vi "XY Graph Get Head & Tail Fraction from Cursors.vi"(5 "Active Plot Index":i32, 6 "Use Cursors":bool, 7 "XYGraph in":T1, 8 "error in (no error)":errorcluster, 9 "Tail Fraction":dbl, 10 "Head Fraction":dbl, 11 "Plot in (Default: Use XY Graph refnum & Plot Id)":cluster{"X Array":dbl[], "Y Array":dbl[]}) -> (0 "error out":errorcluster, 1 "Tail Fraction":dbl, 2 "Head Fraction":dbl, 3 "Plot out":cluster{"X Array":dbl[], "Y Array":dbl[]}, 4 "Plot Name":string)   [LabVIEW 2021, in "XY Graph Add-Ons.lvlib"]
doc: "Computes the fractional location of the head and tail fraction from the <B>HE</B> and <B>TS</B> cursors locations.\n\nIf one (or both) of the cursors is missing, keep the existing values."
uses:
  XY Graph Add-Ons.lvlib
  XY Graph Refnum.ctl
  Strings/Strings.lvlib
  Sound/Sound.lvlib
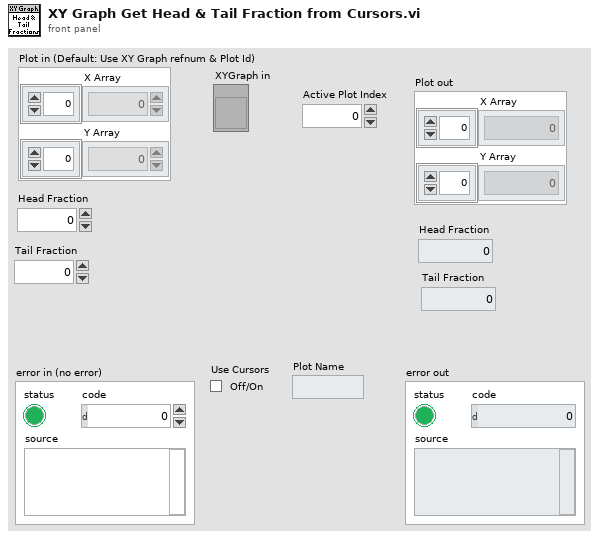
[diagram p1: front panel]
types:
  T1 = typedef "XY Graph Add-Ons.lvlib/XY Graph Refnum.ctl" = refnum<vi>
  T2 = typedef "LVCursorListTypeDef.ctl" = cluster{"Name":string, "Color":u32, "Style":u8, "Point Style":u8, "Name Visible":bool, "Allow Drag":bool, "Cursor Mode":u32, "Plot":i32, "Index":i32, "Position":cluster{"X":dbl, "Y":dbl}, "X Scale":u32, "Y Scale":u32, "Watch Plots":i32[], "Watch All Plots":bool, "Plot Area":i32, "Label Offset":cluster{"X":dbl, "Y":dbl}}[]
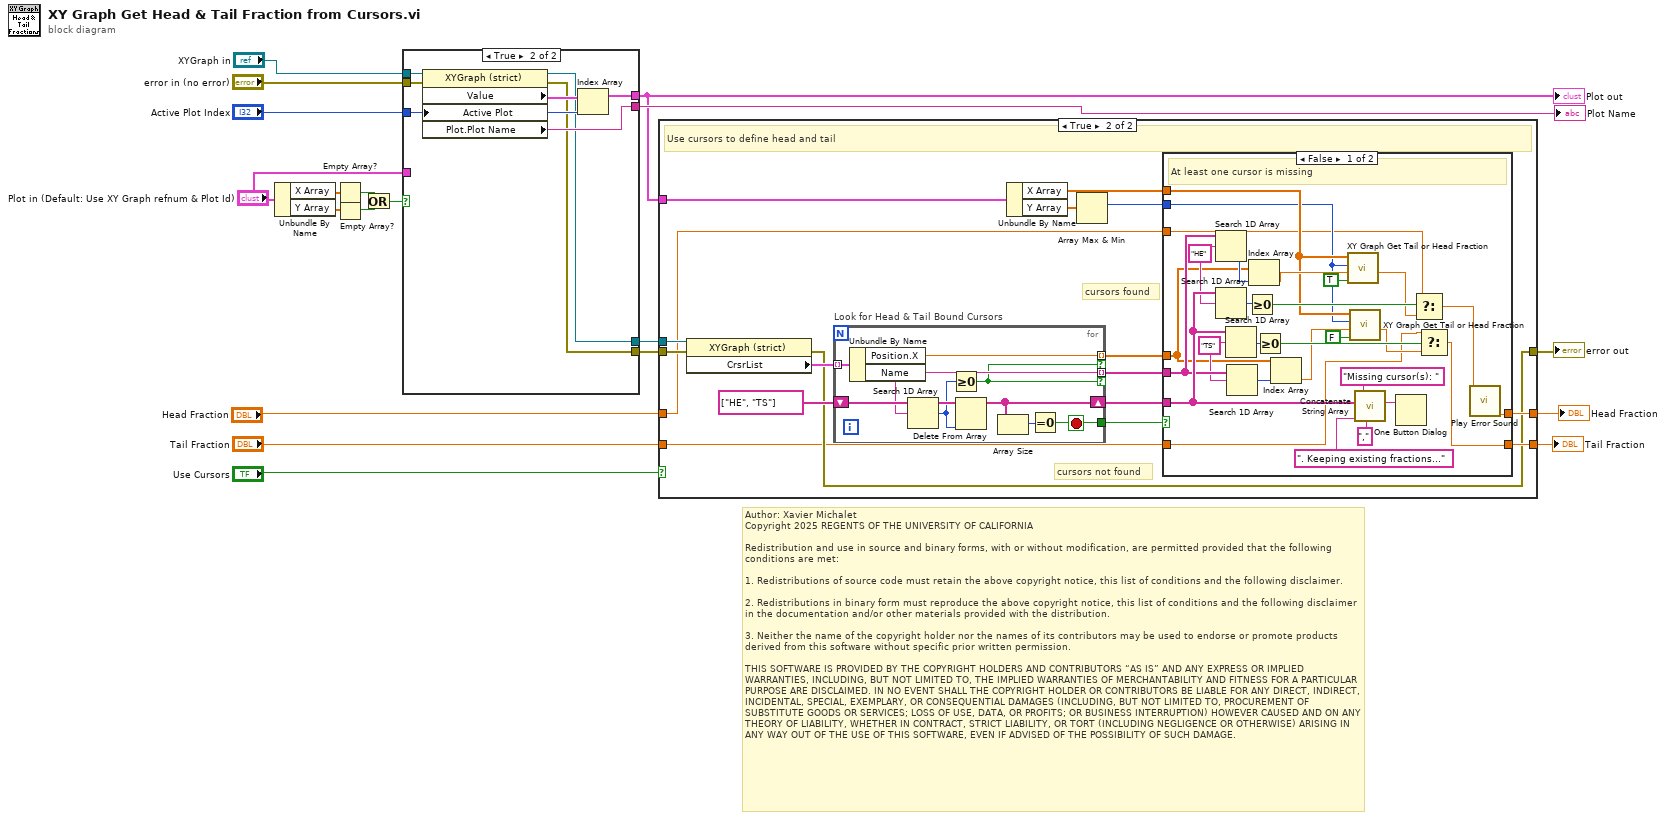
[diagram p0: block diagram]
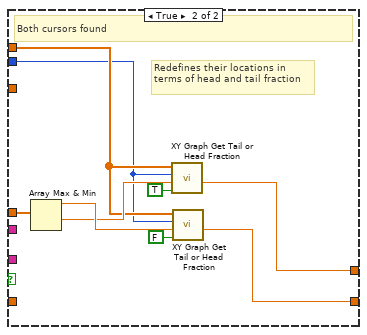
[diagram p4: hidden frame]
diagram:
  # "Author: Xavier Michalet\nCopyright 2025 REGENTS OF THE UNIVERSITY OF CALIFORNIA\n\nRedistribution and use in source and binary forms, with or without modification, are permitted provided that the following conditions are met:\n\n1. Redistributions of source code must retain the above copyright notice, this list of conditions and the following disclaimer.\n\n2. Redistributions in binary form must reproduce the above copyright notice, this list of conditions and the following disclaimer in the documentation and/or other materials provided with the distribution.\n\n3. Neither the name of the copyright holder nor the names of its contributors may be used to endorse or promote products derived from this software without specific prior written permission.\n\nTHIS SOFTWARE IS PROVIDED BY THE COPYRIGHT HOLDERS AND CONTRIBUTORS “AS IS” AND ANY EXPRESS OR IMPLIED WARRANTIES, INCLUDING, BUT NOT LIMITED TO, THE IMPLIED WARRANTIES OF MERCHANTABILITY AND FITNESS FOR A PARTICULAR PURPOSE ARE DISCLAIMED. IN NO EVENT SHALL THE COPYRIGHT HOLDER OR CONTRIBUTORS BE LIABLE FOR ANY DIRECT, INDIRECT, INCIDENTAL, SPECIAL, EXEMPLARY, OR CONSEQUENTIAL DAMAGES (INCLUDING, BUT NOT LIMITED TO, PROCUREMENT OF SUBSTITUTE GOODS OR SERVICES; LOSS OF USE, DATA, OR PROFITS; OR BUSINESS INTERRUPTION) HOWEVER CAUSED AND ON ANY THEORY OF LIABILITY, WHETHER IN CONTRACT, STRICT LIABILITY, OR TORT (INCLUDING NEGLIGENCE OR OTHERWISE) ARISING IN ANY WAY OUT OF THE USE OF THIS SOFTWARE, EVEN IF ADVISED OF THE POSSIBILITY OF SUCH DAMAGE."
  n1 = Unbundle By Name("Plot in (Default: Use XY Graph refnum & Plot Id)") -> ("X Array"=w6:dbl[], "Y Array"=w5:dbl[])
  n2 = Empty Array?(array=w6) -> (empty?=w4:bool)
  n3 = Empty Array?(array=w5) -> (empty?=w3:bool)
  n4 = Or(x=w4, y=w3) -> (x .or. y?=w2:bool)
  n5 = case shown="True" w2 {
    tunnel: "XYGraph in" -> [w20 w30]
    tunnel: "error in (no error)" -> [w21 w29]
    tunnel: "Active Plot Index" -> [_ w27]
    tunnel: [_ w26] -> w16
    tunnel: [w20 w25] -> w11
    tunnel: [w21 w24] -> w10
    tunnel: [w22 w23] -> w9
    tunnel: "Plot in (Default: Use XY Graph refnum & Plot Id)" -> [w22 _]
    frame False {
    }
    frame True {
      n6 = property class="XYGraph (strict)"(reference=w30, error in=w29, "Active Plot"=w27) -> (reference out=w25:T1, error out=w24:errorcluster, "Value"=w28:cluster{"X Array":dbl[], "Y Array":dbl[]}[], "Plot.Plot Name"=w26:string)
      n7 = Index Array(array=w28, index=w27) -> (element=w23:cluster{"X Array":dbl[], "Y Array":dbl[]})
    }
  }
  "Plot out" <- w9
  "Plot Name" <- w16
  n8 = case shown="True" "Use Cursors" {
    tunnel: [w31 w44] -> w14
    tunnel: "Tail Fraction" -> [w33 w34]
    tunnel: [w33 w43] -> w12
    tunnel: w11 -> [_ w50]
    tunnel: w10 -> [w32 w49]
    tunnel: w9 -> [_ w39]
    tunnel: [w32 w41] -> w8
    tunnel: "Head Fraction" -> [w31 w35]
    frame False {
      # "Use percentages to define head and tail"
    }
    frame True {
      # "cursors not found"
      # "cursors found"
      # "Use cursors to define head and tail"
      n9 = property class="XYGraph (strict)"(reference=w50, error in=w49) -> (error out=w41:errorcluster, "CrsrList"=w48:T2)  [unwired: 1 out]
      n10 = for "Look for Head & Tail Bound Cursors" {
        tunnel: w48 -> [w95] mode=indexing
        shift-right: [w93] -> w45
        shift-left: string[] ["HE", "TS"] ("Name") -> [w94]
        tunnel: [w91] -> w42 mode=indexing if=w87
        tunnel: [w89] -> w46
        tunnel: [w88] -> w40 mode=indexing if=w87
        stop <- w89 stop-if-true
        n11 = Unbundle By Name(w95) -> ("Position.X"=w91:dbl, "Name"=w88:string)
        n12 = Search 1D Array(1D array=w94, element=w88) -> (index of element=w90:i32)  [unwired: 1 in]
        n13 = Greater Or Equal To 0?(x=w90) -> (x >= 0?=w87:bool)
        n14 = Delete From Array(array=w94, index=w90) -> (array with subset deleted=w93:string[])  [unwired: 1 in, 1 out]
        n15 = Array Size(array=w93) -> (size(s)=w92:i32)
        n16 = Equal To 0?(x=w92) -> (x = 0?=w89:bool)
      }
      n17 = Unbundle By Name(w39) -> ("X Array"=w38:dbl[], "Y Array"=w37:dbl[])
      n18 = Array Max & Min(array=w37) -> (max index (indices)=w36:i32)  [unwired: 3 out]
      n19 = case shown="False" w46 {
        tunnel: w45 -> [w70 _]
        tunnel: [w71 w81] -> w44
        tunnel: [w67 w80] -> w43
        tunnel: w42 -> [w56 w86]
        tunnel: w40 -> [w65 _]
        tunnel: w38 -> [w59 w79]
        tunnel: w36 -> [w53 w78]
        tunnel: w35 -> [w52 _]
        tunnel: w34 -> [w51 _]
        frame False {
          w64 = "TS" ("element")
          w66 = "HE" ("element")
          # "At least one cursor is missing"
          n20 = Search 1D Array(1D array=w65, element=w66) -> (index of element=w63:i32)  [unwired: 1 in]
          n21 = Search 1D Array(1D array=w70, element=w66) -> (index of element=w73:i32)  [unwired: 1 in]
          n22 = Search 1D Array(1D array=w70, element=w64) -> (index of element=w69:i32)  [unwired: 1 in]
          n23 = Search 1D Array(1D array=w65, element=w64) -> (index of element=w55:i32)  [unwired: 1 in]
          n24 = Greater Or Equal To 0?(x=w73) -> (x >= 0?=w72:bool)
          n25 = Index Array(array=w56, index=w63) -> (element=w62:dbl)
          n26 = Greater Or Equal To 0?(x=w69) -> (x >= 0?=w68:bool)
          n27 = Index Array(array=w56, index=w55) -> (element=w54:dbl)
          n28 = call "XY Graph Get Tail or Head Fraction.vi"("Tail (F)/Head (T)"=TRUE, "Array Index"=w62, "Peak Index"=w53, "X Array"=w59) -> ("Head or Tail Fraction"=w61:dbl)  [unwired: 7 in]
          n29 = call "XY Graph Get Tail or Head Fraction.vi"("Tail (F)/Head (T)"=FALSE, "Array Index"=w54, "Peak Index"=w53, "X Array"=w59) -> ("Head or Tail Fraction"=w57:dbl)  [unwired: 7 in]
          n30 = call "Concatenate String Array.vi"("Separator (TAB)"=",", "Suffix (\"\")"=". Keeping existing fractions..." ("Suffix (\"\")"), "String Array"=w70, "Prefix (\"\")"="Missing cursor(s): " ("Prefix (\"\")")) -> ("Formatted String"=w74:string)  [unwired: 7 in]
          n31 = One Button Dialog(message=w74) -> ()  [unwired: 1 in, 1 out]
          n32 = Select(t=w52, s=w72, f=w61) -> (s? t:f=w71:dbl)
          n33 = Select(t=w51, s=w68, f=w57) -> (s? t:f=w67:dbl)
          n34 = call "Play Error Sound.vi"() -> ()  [unwired: 27 in, 1 out]
        }
        frame True {
          # "Redefines their locations in terms of head and tail fraction"
          # "Both cursors found"
          n35 = Array Max & Min(array=w86) -> (max value=w85:dbl, min value=w83:dbl)  [unwired: 2 out]
          n36 = call "XY Graph Get Tail or Head Fraction.vi"("Tail (F)/Head (T)"=TRUE, "Array Index"=w83, "Peak Index"=w78, "X Array"=w79) -> ("Head or Tail Fraction"=w81:dbl)  [unwired: 7 in]
          n37 = call "XY Graph Get Tail or Head Fraction.vi"("Tail (F)/Head (T)"=FALSE, "Array Index"=w85, "Peak Index"=w78, "X Array"=w79) -> ("Head or Tail Fraction"=w80:dbl)  [unwired: 7 in]
        }
      }
    }
  }
  "error out" <- w8
  "Head Fraction" <- w14
  "Tail Fraction" <- w12
